vi "Read System Name.vi"(8 "error in (no error)":errorcluster, 11 "crio configuration in":refnum<class "crio configuration.lvclass">) -> (0 "error out":errorcluster, 2 "System Name":string, 3 "crio configuration out":refnum<class "crio configuration.lvclass">)   [LabVIEW 2013, in "crio configuration.lvclass"]
uses:
  crio configuration.lvclass
  CEF_TreeControl/serializable configuration/NISE_CEF_serializable configuration.lvclass
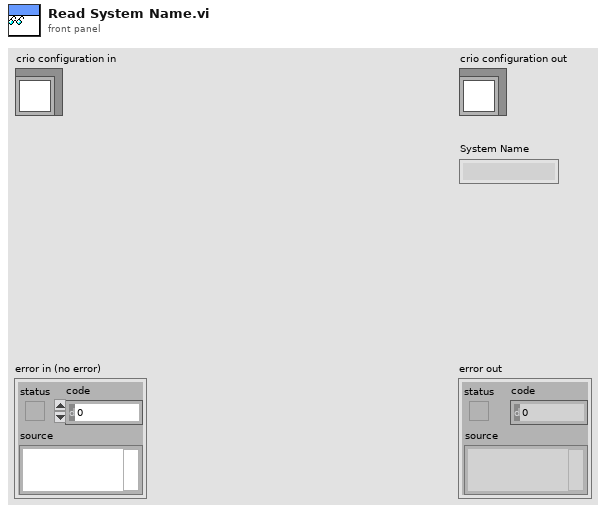
[diagram p1: front panel]
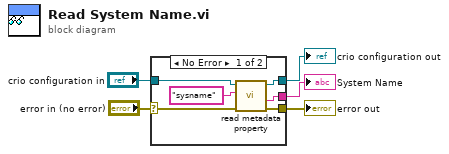
[diagram p0: block diagram]
diagram:
  n1 = case shown="No Error" "error in (no error)" {
    selector: "error in (no error)" -> [w9 w12]
    tunnel: [w8 w12] -> w4
    tunnel: [w10 w13] -> w2
    tunnel: "crio configuration in" -> [w11 w13]
    tunnel: [w7 _] -> w1
    frame No Error {
      n2 = call "read metadata property.vi"("error in"=w9, "key"="sysname", "configuration in"=w11) -> ("error out"=w8:errorcluster, "value"=w7:string, "configuration out"=w10:refnum<class "crio configuration.lvclass">)  [unwired: 5 in, 1 out]
    }
    frame Error {
    }
  }
  "error out" <- w4
  "crio configuration out" <- w2
  "System Name" <- w1
